vi "reg-log-irr.vi"(6 "Operation(Read)":T3, 8 "error in":errorcluster, 9 "Rows":i32=20, 10 "filter by proc name":cluster{"ProcName":string, "StepIndex":i32}={"ProcName"="", "StepIndex"=-1}, 11 "Reports to Collect":T4 {"clk" format="%#.3f"}) -> (0 "error out":errorcluster, 2 "compact report":T1[](array[typedef]) {"clk" format="%#.1f"}, 3 "Collected Reports":T4[](array[typedef]) {"clk" format="%#.3f"})   [LabVIEW 2024]
uses:
  controls/typeEngineLogCluster.ctl
  controls/type.StepFunction.ctl
  controls/enum.report-filter.ctl
  controls/UiCompactReport.ctl
panel:
  out "size(s)":i32
  # "stepIndex>=0 then filter by step index\nstepIndex==-1 then do not filter"
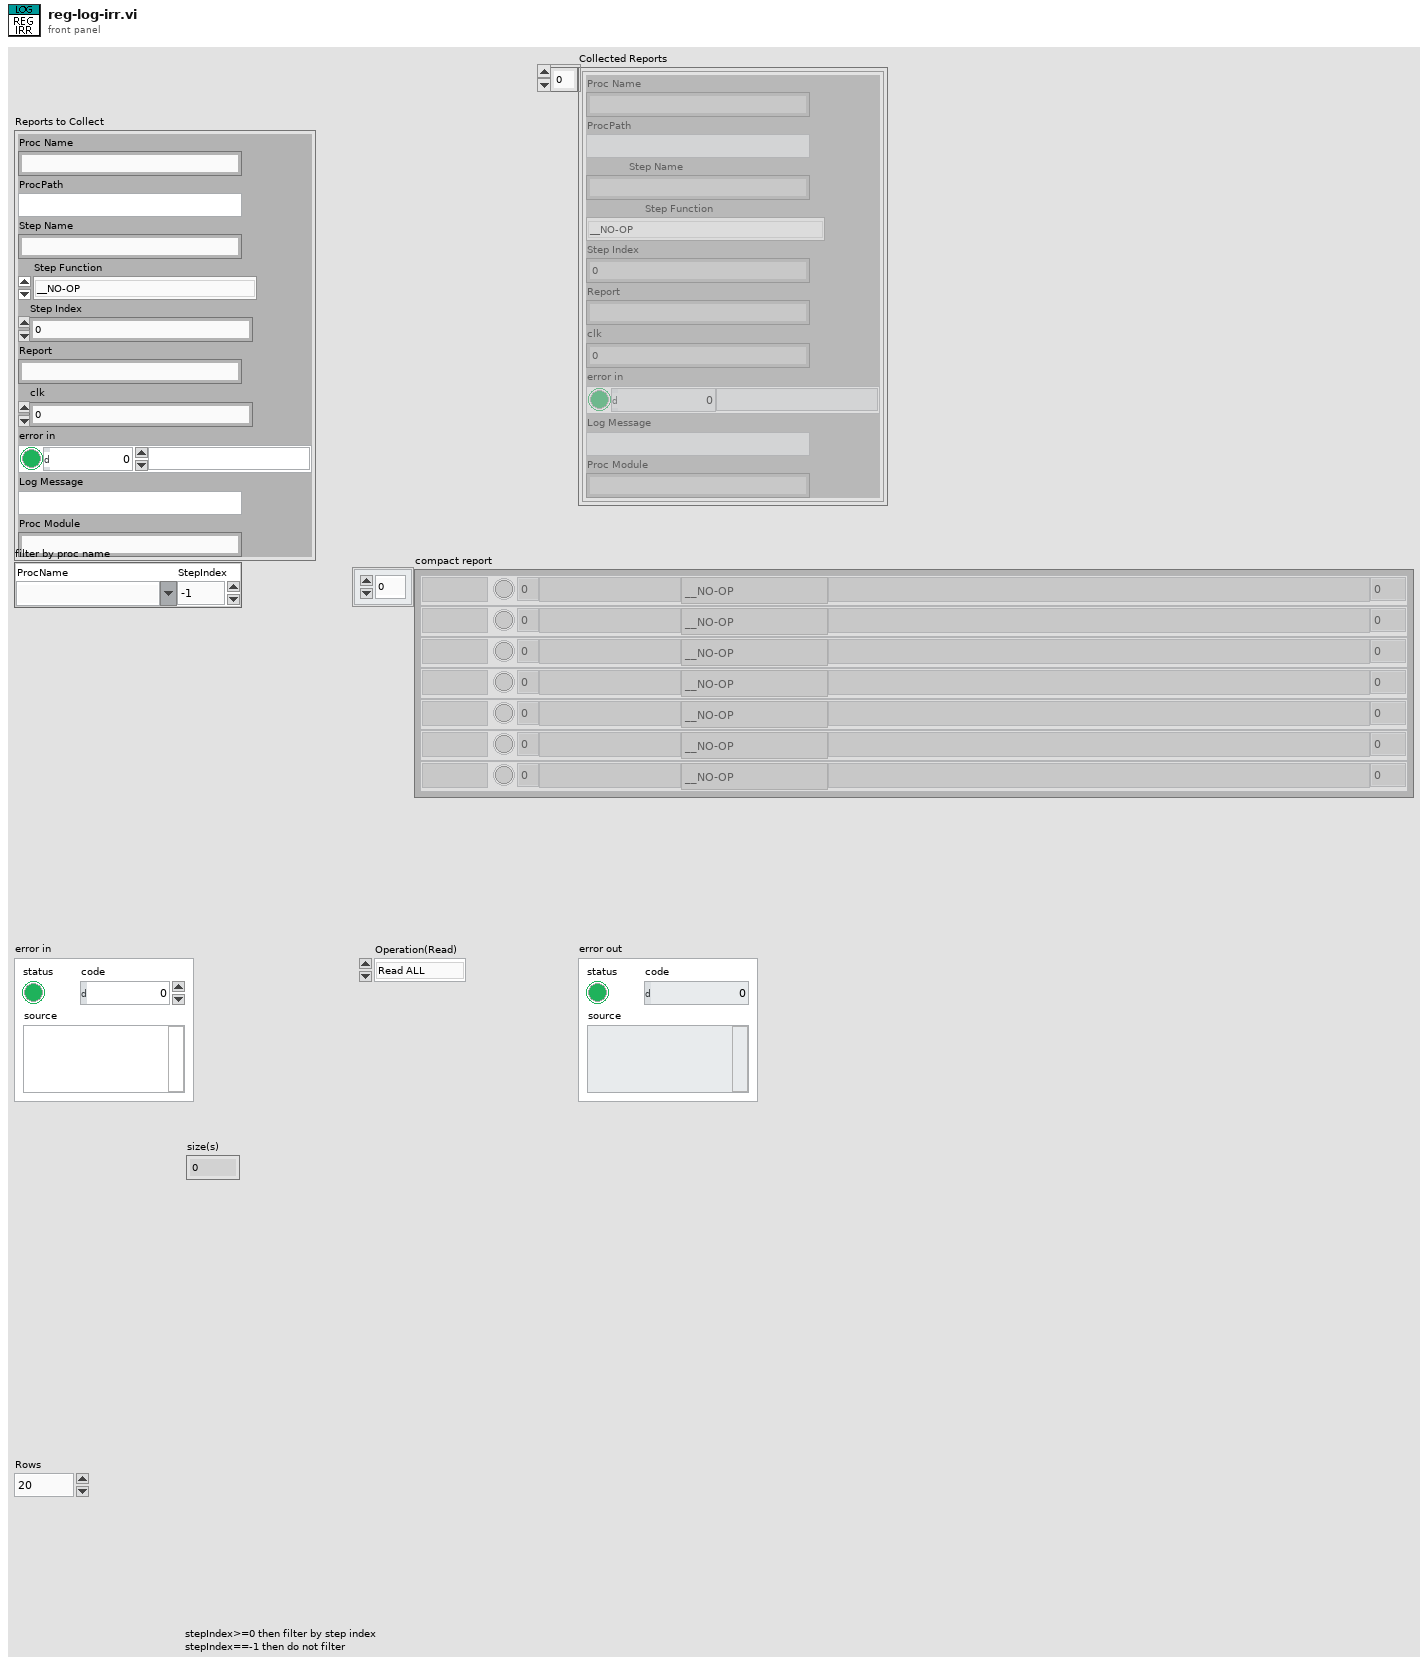
[diagram p1: front panel]
types:
  T1 = typedef "UiCompactReport.ctl" = cluster{"ErrorFlag":bool, "idx":i32, "Step Name":string, "Step Function":T2, "Report":string, "clk":dbl, "Proc":string}
  T2 = typedef "type.StepFunction.ctl" = enum16{"__NO-OP", "_DELAY_LOAD", "_DELAY_COMPARE", "_JUMP", "_COMPLETE", "_COMPARE", "_LOG_MESSAGE", "_LOG_LAST_REPORT", "_SCHEDULE", "_SCHED_DAILY", "CLK_COMPARE", "PROC_START", "PROC_STOP", "PROC_LOAD", "PROC_COMPLETION_CHECK", "PROC_COMPLETION_LOAD", "_IO_READ", "_IO_READ_MANY", "_IO_WRITE", "_IO_WRITE_BY_REG", "_IO_GET_OUTPUT", "_OCS_CHECK", "_OCS_RECORD", "_GET_RH", "_GET_ACC_UV", "_GET_WD", "_GET_WS", "_REC_DELETE", "_REC_MOVE", "_REC_COPY", "_IRR_CHECK", "UNIT_CHECK", "UNIT_SAMPLE", "UNIT_DOSE"}
  T3 = typedef "enum.report-filter.ctl" = enum16{"Read ALL", "Read Errors", "Collect", "ClearAll"}
  T4 = typedef "typeEngineLogCluster.ctl" = cluster{"Proc Name":string, "ProcPath":string, "Step Name":string, "Step Function":T2, "Step Index":i32, "Report":string, "clk":dbl, "error in":errorcluster, "Log Message":string, "Proc Module":string}
  T5 = cluster{"Proc Name":bool, "ProcPath":bool, "Step Name":bool, "Step Function":bool, "Step Index":bool, "Report":bool, "clk":bool, "error in":cluster{"status":bool, "code":bool, "source":bool}, "Log Message":bool, "Proc Module":bool}
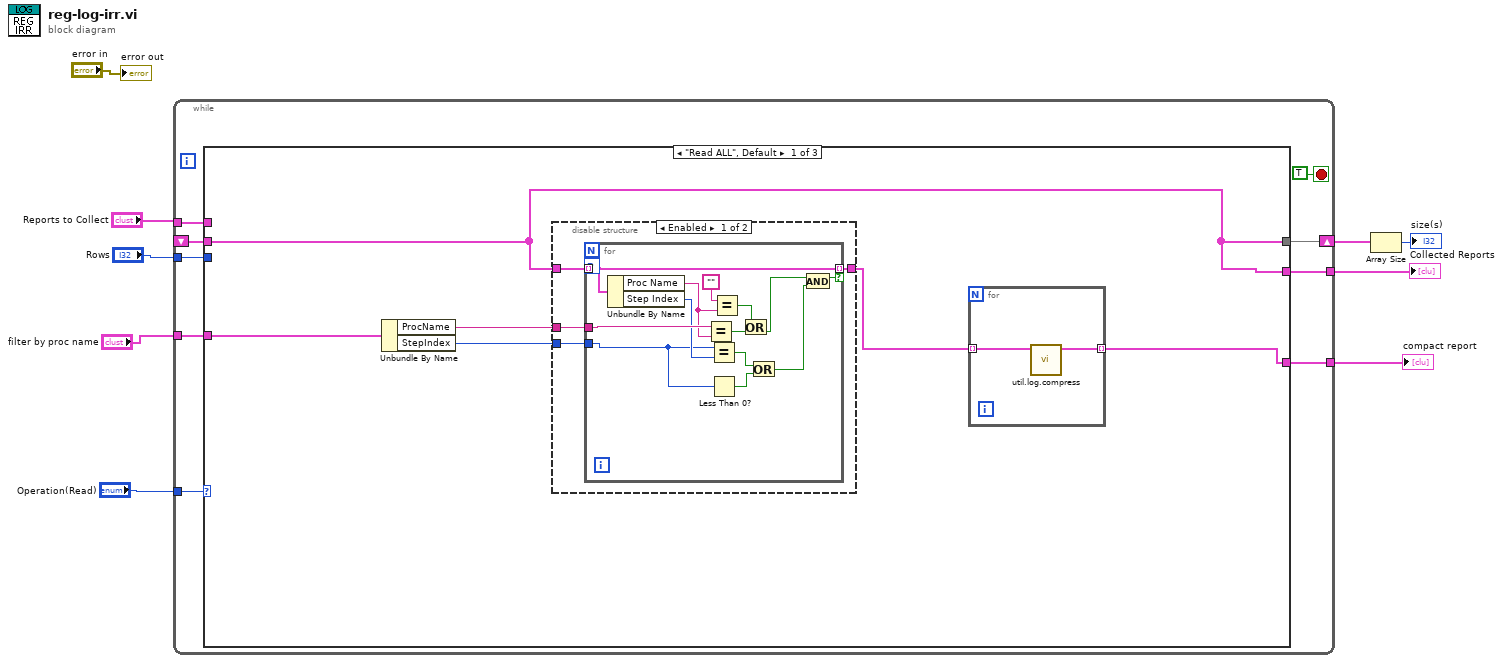
[diagram p0: block diagram]
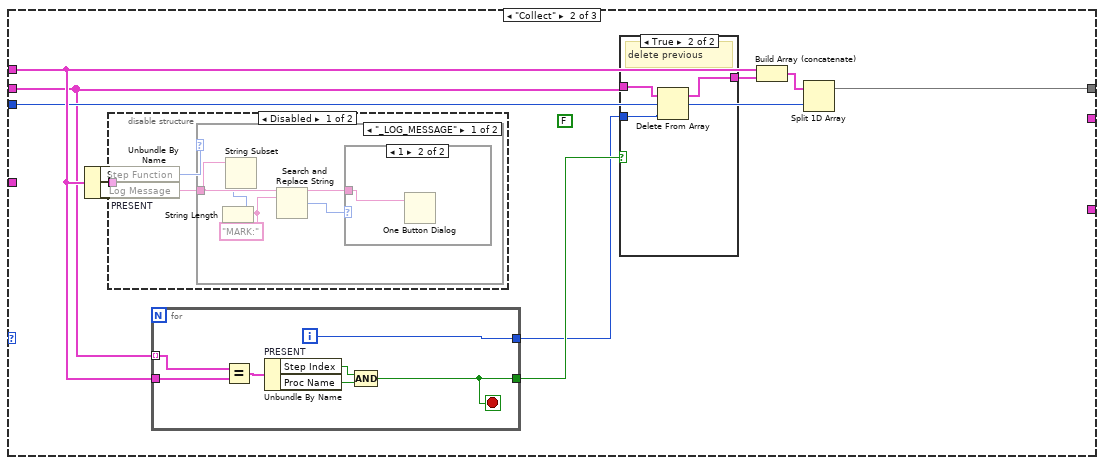
[diagram p3: hidden frame]
diagram:
  n1 = while {
    shift-right: [w16] -> w6
    shift-left: _ -> [w14]
    tunnel: "Reports to Collect" -> [w18]
    tunnel: "Rows" -> [w15]
    tunnel: "Operation(Read)" -> [w13]
    tunnel: [w12] -> w4
    tunnel: [w11] -> w3
    tunnel: "filter by proc name" -> [w10]
    stop <- TRUE stop-if-true
    n2 = case shown="\"Read ALL\", Default" w13 {
      tunnel: w18 -> [_ w52 _]
      tunnel: [w24 w51 _] -> w16
      tunnel: w15 -> [_ w50 _]
      tunnel: w14 -> [w24 w49 _]
      tunnel: [w24 _ _] -> w12
      tunnel: [w21 _ _] -> w11
      tunnel: w10 -> [w20 _ _]
      frame "Read ALL", Default {
        n3 = Unbundle By Name(w20) -> ("ProcName"=w23:string, "StepIndex"=w22:i32)
        n4 = disable-structure shown="Enabled" {
          disable-tunnel: w24 -> [w30 w44]
          disable-tunnel: w23 -> [w29 _]
          disable-tunnel: w22 -> [w28 _]
          disable-tunnel: [w27 w44] -> w19
          frame Enabled {
            n5 = for {
              tunnel: w30 -> [w31] mode=indexing
              tunnel: w29 -> [w42]
              tunnel: [w31] -> w27 mode=indexing if=w37
              tunnel: w28 -> [w40]
              workers-P: _ -> [_]
              n6 = Unbundle By Name(w31) -> ("Proc Name"=w34:string, "Step Index"=w41:i32)
              n7 = Equal?(x=w42, y=w34) -> (x = y?=w43:bool)
              n8 = Equal?(x=w40, y=w41) -> (x = y?=w39:bool)
              n9 = Less Than 0?(x=w40) -> (x < 0?=w38:bool)
              n10 = Equal?(x="", y=w34) -> (x = y?=w32:bool)
              n11 = Or(x=w32, y=w43) -> (x .or. y?=w35:bool)
              n12 = Or(x=w39, y=w38) -> (x .or. y?=w36:bool)
              n13 = And(x=w35, y=w36) -> (x .and. y?=w37:bool)
            }
          }
          frame Disabled {
          }
        }
        n14 = for {
          tunnel: [w26] -> w21 mode=indexing
          tunnel: w19 -> [w25] mode=indexing
          n15 = call "util.log.compress.vi"("Log Cluster in"=w25) -> ("Compact Report"=w26:T1)  [unwired: 9 in, 1 out]
        }
      }
      frame "Collect" {
        (unwired) FALSE
        n16 = disable-structure shown="Disabled" {
          disable-tunnel: w52 -> [w62 _]
          frame Disabled {
            n17 = Unbundle By Name "PRESENT"(w62) -> ("Step Function"=w60:T2, "Log Message"=w61:string)
            n18 = case shown="\"_LOG_MESSAGE\"" w60 {
              tunnel: w61 -> [w66 _]
              frame "_LOG_MESSAGE" {
                w64 = "MARK:" ("search string")
                n19 = String Length(string=w64) -> (length=w65:i32)
                n20 = String Subset(string=w66, length (rest)=w65) -> ()  [unwired: 1 in, 1 out]
                n21 = Search and Replace String(input string=w66, search string=w64) -> (result string=w63:string, number of replacements=w67:i32)  [unwired: 6 in, 2 out]
                n22 = case shown="1" w67 {
                  tunnel: w63 -> [_ w68]
                  frame 0, Default {
                  }
                  frame 1 {
                    n23 = One Button Dialog(message=w68) -> ()  [unwired: 1 in, 1 out]
                  }
                }
              }
              frame Default {
              }
            }
          }
          frame Enabled {
          }
        }
        n24 = for {
          tunnel: w52 -> [w59]
          tunnel: w49 -> [w58] mode=indexing
          tunnel: [w54] -> w46
          tunnel: [w53] -> w45
          i -> [w53]
          stop <- w54 stop-if-true
          n25 = Equal?(x=w58, y=w59) -> (x = y?=w57:T5)
          n26 = Unbundle By Name "PRESENT"(w57) -> ("Step Index"=w55:bool, "Proc Name"=w56:bool)
          n27 = Compound Arithmetic op=AND(w55, w56) -> (w54:bool)
        }
        n28 = case shown="True" w46 {
          tunnel: w49 -> [w69 w72]
          tunnel: [w69 w71] -> w48
          tunnel: w45 -> [_ w70]
          frame False {
          }
          frame True {
            # "delete previous"
            n29 = Delete From Array(array=w72, index=w70) -> (array with subset deleted=w71:T4[])  [unwired: 1 in, 1 out]
          }
        }
        n30 = Build Array (concatenate)(w52, w48) -> (w47:T4[])
        n31 = Split 1D Array(array=w47, index=w50) -> (first subarray=w51:T4[])  [unwired: 1 out]
      }
      frame "ClearAll" {
      }
    }
  }
  "Collected Reports" <- w4
  "compact report" <- w3
  n32 = Array Size(array=w6) -> (size(s)=→"size(s)":i32)
  "error out" <- "error in"
